vi "Post Initialize Action.vi"(8 "error in (no error)":errorcluster, 11 "Helper Methods in":refnum<class "Helper Methods.lvclass">) -> (0 "error out":errorcluster, 2 "Init Event Data":variant, 3 "Helper Methods out":refnum<class "Helper Methods.lvclass">)   [LabVIEW 2017, in "2. Basic Panel Actors.lvlib" / "Helper Methods.lvclass"]
doc: "This VI is called just after the Panel Actor's UI was initialized.\n\nData wired to <b>Init Event Data</b> will be passed in the panel's \"Initialized\" user event.\n\nIf there were any initialization errors they should be handled here.\n----\nCopyright: MGI 2016\nAuthor: Derek Trepanier"
uses:
  Helper Methods.lvclass
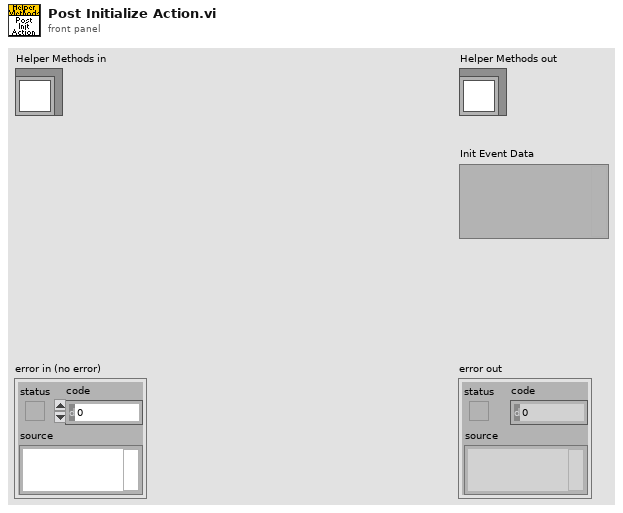
[diagram p1: front panel]
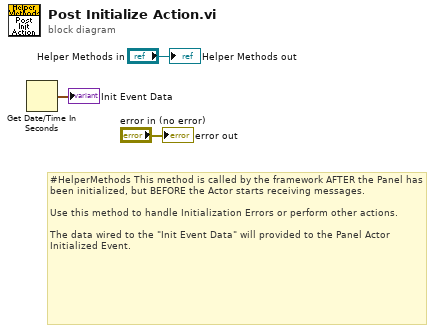
[diagram p0: block diagram]
diagram:
  # "#HelperMethods This method is called by the framework AFTER the Panel has been initialized, but BEFORE the Actor starts receiving messages.\n\nUse this method to handle Initialization Errors or perform other actions.\n\nThe data wired to the \"Init Event Data\" will provided to the Panel Actor Initialized Event."
  n1 = Get Date/Time In Seconds() -> (seconds since 1Jan1904=→"Init Event Data":timestamp)
  "error out" <- "error in (no error)"
  "Helper Methods out" <- "Helper Methods in"
